vi "System Config - format and values.vi"(11 "System Config":T4={"Laser wavelength (nm)"=920.0, "DAQ FPGA System"={"Clock Freq (MHz) "=200.0, "Samples Wait after Trigger"=5080, "AOD fill"=4900, "StartupDelay"=0, "Slip Cycle (clock cycles)"=600000, "Add Cycle"=TRUE}, "Control system"={"AOD 1 Amplitude"=0, "AOD 2 Amplitude"=0, "AOD 3 Amplitude"=0, "AOD 4 Amplitude"=0, "AOD 5 Amplitude"=0, "AOD 6 Amplitude"=0, "T0 (ns)"=0.0, "Ta (ns)"=0.0, "Data Time Interval (ns)"=0.0, "Ctrl FPGA Clock (MHz)"=240.0}} {"Control system"."Ctrl FPGA Clock (MHz)" min=80.0 max=500.0 step=1.0; "Control system"."Data Time Interval (ns)" min=0.0 max=2048.0 step=1.0; "Control system"."Ta (ns)" min=0.0 max=2048.0 step=1.0; "Control system"."T0 (ns)" min=0.0 max=2048.0 step=1.0; "Control system"."AOD 6 Amplitude" min=0 max=2048 step=1; "Control system"."AOD 5 Amplitude" min=0 max=2048 step=1; "Control system"."AOD 4 Amplitude" min=0 max=2048 step=1; "Control system"."AOD 3 Amplitude" min=0 max=2048 step=1; "Control system"."AOD 2 Amplitude" min=0 max=2048 step=1; "Control system"."AOD 1 Amplitude" min=0 max=2048 step=1; "Laser wavelength (nm)" min=800.0 max=1080.0 step=1.0}) -> (0 "String Values":string[](array[string]), 1 "String":T1(array[cluster]), 2 "Numeric Values":dbl[](array[numeric]), 3 "Numeric":T3=[{"key"="Control system.Clock freq (MHz)", "Save?"=TRUE, "Default"=240.0}, {"key"="DAQ FPGA.Clock freq (MHz)", "Save?"=TRUE, "Default"=200.0}, {"key"="Control system.AOD 1 Amplitude", "Save?"=TRUE, "Default"=0.0}, {"key"="Control system.AOD 2 Amplitude", "Save?"=TRUE, "Default"=0.0}, {"key"="Control system.AOD 3 Amplitude", "Save?"=TRUE, "Default"=0.0}, {"key"="Control system.AOD 4 Amplitude", "Save?"=TRUE, "Default"=0.0}, {"key"="Control system.AOD 5 Amplitude", "Save?"=TRUE, "Default"=0.0}, {"key"="Control system.AOD 6 Amplitude", "Save?"=TRUE, "Default"=0.0}, {"key"="Control system.Data Time Interval (ns)", "Save?"=TRUE, "Default"=50.0}, {"key"="Control system.T0 (ns)", "Save?"=TRUE, "Default"=0.0}, {"key"="Control system.Ta (ns)", "Save?"=TRUE, "Default"=0.0}, {"key"="Laser wavelength (nm)", "Save?"=TRUE, "Default"=800.0}, {"key"="DAQ FPGA.Samples Wait after Trigger", "Save?"=TRUE, "Default"=5080.0}, {"key"="DAQ FPGA.AOD fill", "Save?"=TRUE, "Default"=4900.0}, {"key"="DAQ FPGA.StartupDelay", "Save?"=TRUE, "Default"=0.0}, {"key"="DAQ FPGA.Slip Cycle", "Save?"=TRUE, "Default"=400000.0}], 4 "Boolean Values":bool[](array[boolean]), 6 "Boolean":T2(array[cluster])=[{"key"="DAQ FPGA.Add Cycle", "Save?"=FALSE, "Default"=TRUE}])   [LabVIEW 2020]
uses:
  Typedefs/System Configuration.ctl
  Typedefs/DAQ FPGA system config.ctl
  Typedefs/CTRL system config.ctl
  Typedefs/Ini file interface (DBL).ctl
panel:
  out "Numeric Size":i32
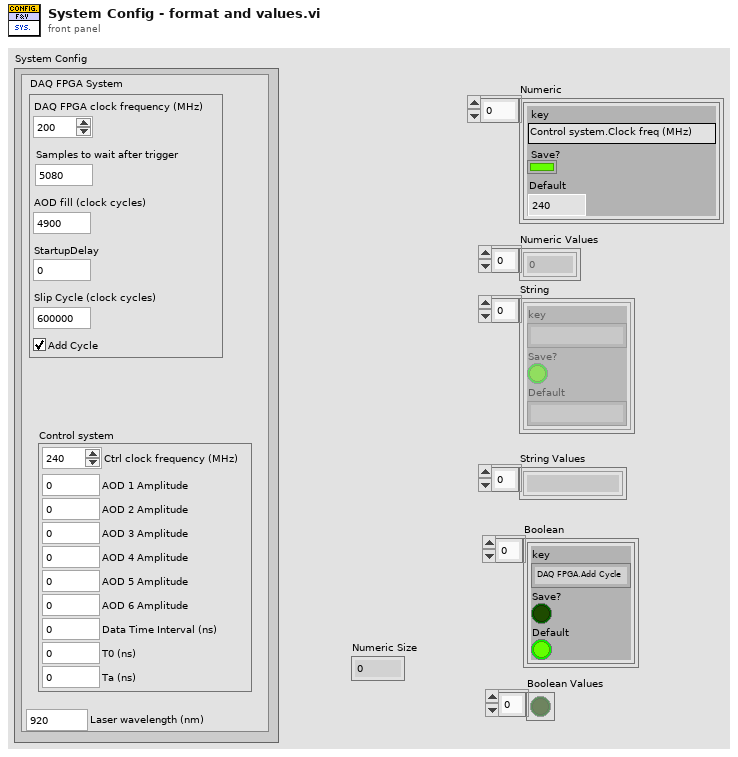
[diagram p1: front panel]
types:
  T1 = cluster{"key":string, "Save?":bool, "Default":string}[]
  T2 = cluster{"key":string, "Save?":bool, "Default":bool}[]
  T3 = typedef "Ini file interface (DBL).ctl" = cluster{"key":string, "Save?":bool, "Default":dbl}[]
  T4 = typedef "System Configuration.ctl" = cluster{"Laser wavelength (nm)":dbl, "DAQ FPGA System":T5, "Control system":T6}
  T5 = typedef "DAQ FPGA system config.ctl" = cluster{"Clock Freq (MHz) ":dbl, "Samples Wait after Trigger":u16, "AOD fill":u16, "StartupDelay":i32, "Slip Cycle (clock cycles)":u32, "Add Cycle":bool}
  T6 = typedef "CTRL system config.ctl" = cluster{"AOD 1 Amplitude":i16, "AOD 2 Amplitude":i16, "AOD 3 Amplitude":i16, "AOD 4 Amplitude":i16, "AOD 5 Amplitude":i16, "AOD 6 Amplitude":i16, "T0 (ns)":dbl, "Ta (ns)":dbl, "Data Time Interval (ns)":dbl, "Ctrl FPGA Clock (MHz)":dbl}
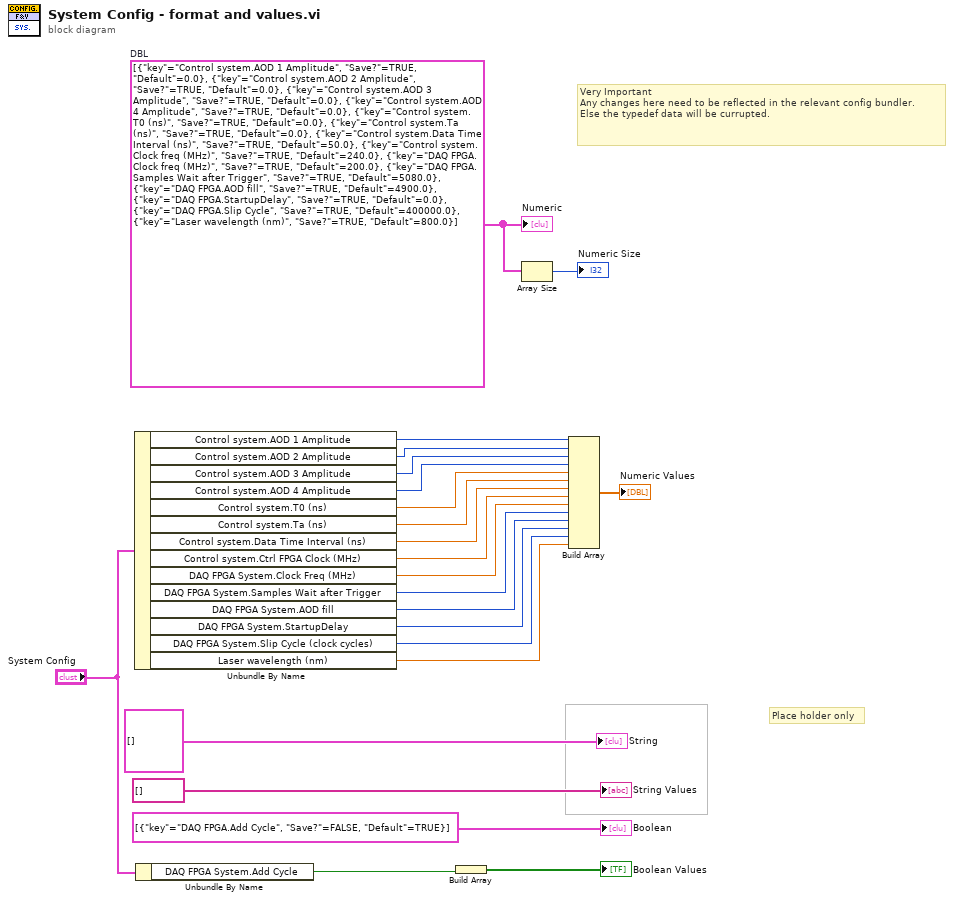
[diagram p0: block diagram]
diagram:
  w22 = T3 [{"key"="Control system.AOD 1 Amplitude", "Save?"=TRUE, "Default"=0.0}, {"key"="Control system.AOD 2 Amplitude", "Save?"=TRUE, "Default"=0.0}, {"key"="Control system.AOD 3 Amplitude", "Save?"=TRUE, "Default"=0.0}, {"key"="Control system.AOD 4 Amplitude", "Save?"=TRUE, "Default"=0.0}, {"key"="Control system.T0 (ns)", "Save?"=TRUE, "Default"=0.0}, {"key"="Control system.Ta (ns)", "Save?"=TRUE, "Default"=0.0}, {"key"="Control system.Data Time Interval (ns)", "Save?"=TRUE, "Default"=50.0}, {"key"="Control system.Clock freq (MHz)", "Save?"=TRUE, "Default"=240.0}, {"key"="DAQ FPGA.Clock freq (MHz)", "Save?"=TRUE, "Default"=200.0}, {"key"="DAQ FPGA.Samples Wait after Trigger", "Save?"=TRUE, "Default"=5080.0}, {"key"="DAQ FPGA.AOD fill", "Save?"=TRUE, "Default"=4900.0}, {"key"="DAQ FPGA.StartupDelay", "Save?"=TRUE, "Default"=0.0}, {"key"="DAQ FPGA.Slip Cycle", "Save?"=TRUE, "Default"=400000.0}, {"key"="Laser wavelength (nm)", "Save?"=TRUE, "Default"=800.0}]  # DBL
  # "Very Important\nAny changes here need to be reflected in the relevant config bundler.\nElse the typedef data will be currupted."
  # "Place holder only"
  n1 = Unbundle By Name("System Config") -> ("Control system.AOD 1 Amplitude"=w19:i16, "Control system.AOD 2 Amplitude"=w18:i16, "Control system.AOD 3 Amplitude"=w17:i16, "Control system.AOD 4 Amplitude"=w16:i16, "Control system.T0 (ns)"=w15:dbl, "Control system.Ta (ns)"=w14:dbl, "Control system.Data Time Interval (ns)"=w13:dbl, "Control system.Ctrl FPGA Clock (MHz)"=w12:dbl, "DAQ FPGA System.Clock Freq (MHz)"=w11:dbl, "DAQ FPGA System.Samples Wait after Trigger"=w10:u16, "DAQ FPGA System.AOD fill"=w9:u16, "DAQ FPGA System.StartupDelay"=w8:i32, "DAQ FPGA System.Slip Cycle (clock cycles)"=w7:u32, "Laser wavelength (nm)"=w6:dbl)
  n2 = Unbundle By Name("System Config") -> ("DAQ FPGA System.Add Cycle"=w4:bool)
  n3 = Build Array(w4) -> (→"Boolean Values":bool[])
  n4 = Array Size(array=w22) -> (size(s)=→"Numeric Size":i32)
  n5 = Build Array(w19, w18, w17, w16, w15, w14, w13, w12, w11, w10, w9, w8, w7, w6) -> (→"Numeric Values":dbl[])
  "Numeric" <- w22
  "Boolean" <- T2 [{"key"="DAQ FPGA.Add Cycle", "Save?"=FALSE, "Default"=TRUE}]
  "String Values" <- string[] []
  "String" <- T1 [] ("Ini file interface (String)")
